vi "Calib_and_iRFAlign_confirm.vi"(6 "Current V":T1, 8 "Ch4 Data":dbl[][](array[numeric]), 9 "Ch3 Data":dbl[][](array[numeric]), 10 "Ch2 Data":dbl[][](array[numeric]), 11 "Ch1 Data":dbl[][](array[numeric])) -> (2 "Save?":bool)   [LabVIEW 2020]
uses:
  GlobalVariables.vi
panel:
  out "Reference Gain":dbl format="%#_3g"
  out "Gain4":dbl format="%#_3g"
  out "Reference V4":dbl format="%#_4g"
  out "Channel 4":dbl[][](graph)
  out "V4":dbl format="%#_4g"
  out "Reference Gain3":dbl format="%#_3g"
  out "Reference Gain 2":dbl format="%#_3g"
  out "Gain3":dbl format="%#_3g"
  out "Gain2":dbl format="%#_3g"
  out "Gain1":dbl format="%#_3g"
  out "Reference Gian1":dbl format="%#_3g"
  out "Reference V3":dbl format="%#_4g"
  out "Reference V2":dbl format="%#_4g"
  out "Reference V1":dbl format="%#_4g"
  in  "Cancel Button":bool
  in  "Save Button":bool
  out "Channel 3":dbl[][](graph)
  out "Channel 2":dbl[][](graph)
  out "Channel 1":dbl[][](graph)
  out "V3":dbl format="%#_4g"
  out "V2":dbl format="%#_4g"
  out "V1":dbl format="%#_4g"
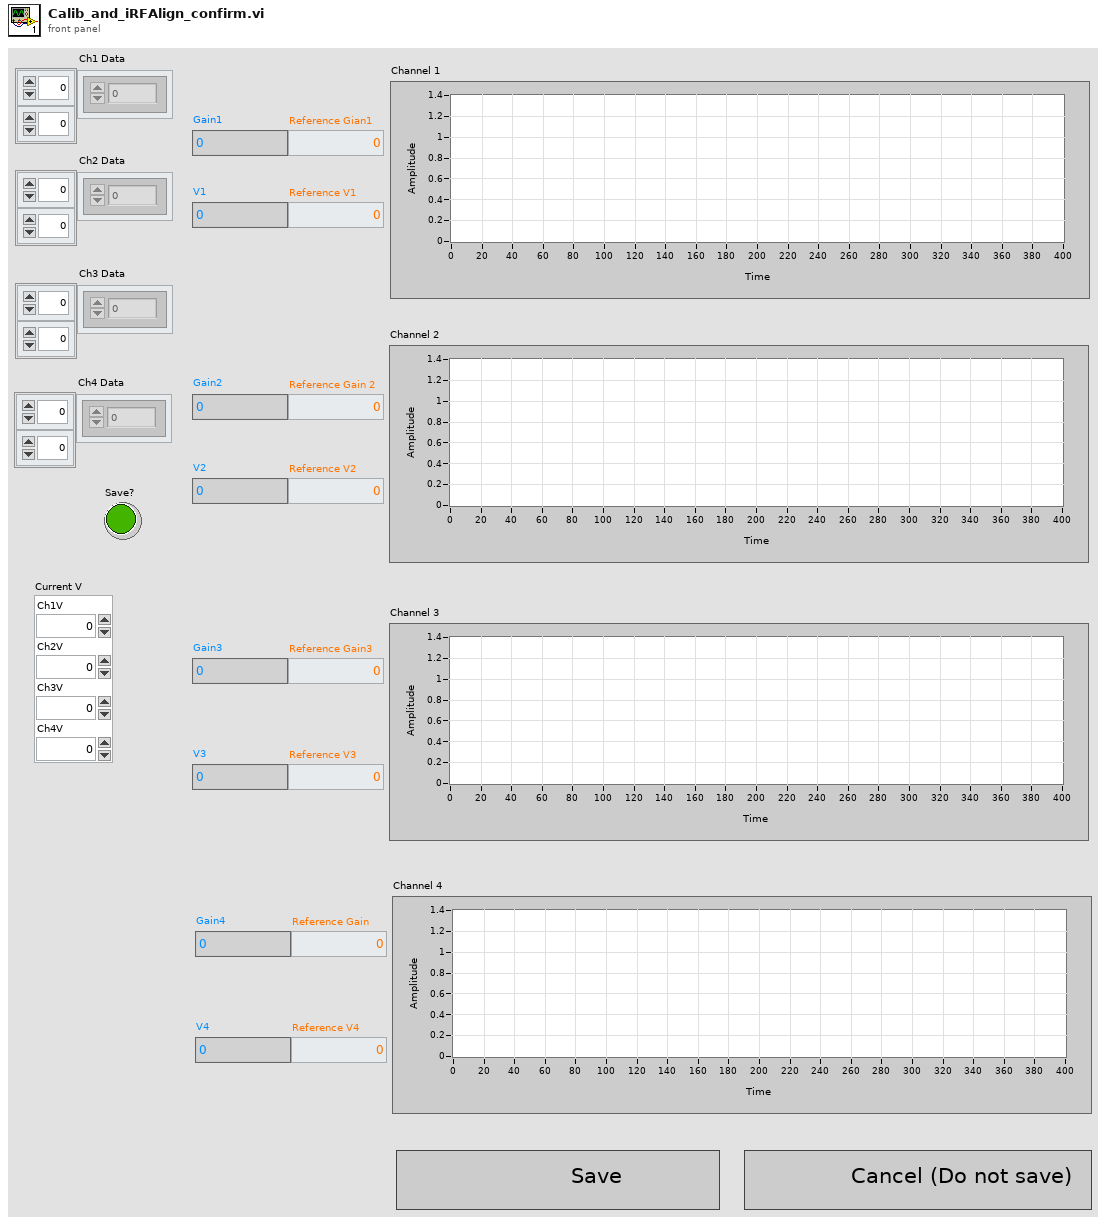
[diagram p1: front panel]
types:
  T1 = cluster{"Ch1V":dbl, "Ch2V":dbl, "Ch3V":dbl, "Ch4V":dbl}
  T2 = cluster{"Ch1 WF":dbl[], "Ch2 WF":dbl[], "Ch3 WF":dbl[], "Ch4 WF":dbl[], "V1":dbl, "V2":dbl, "V3":dbl, "V4":dbl}
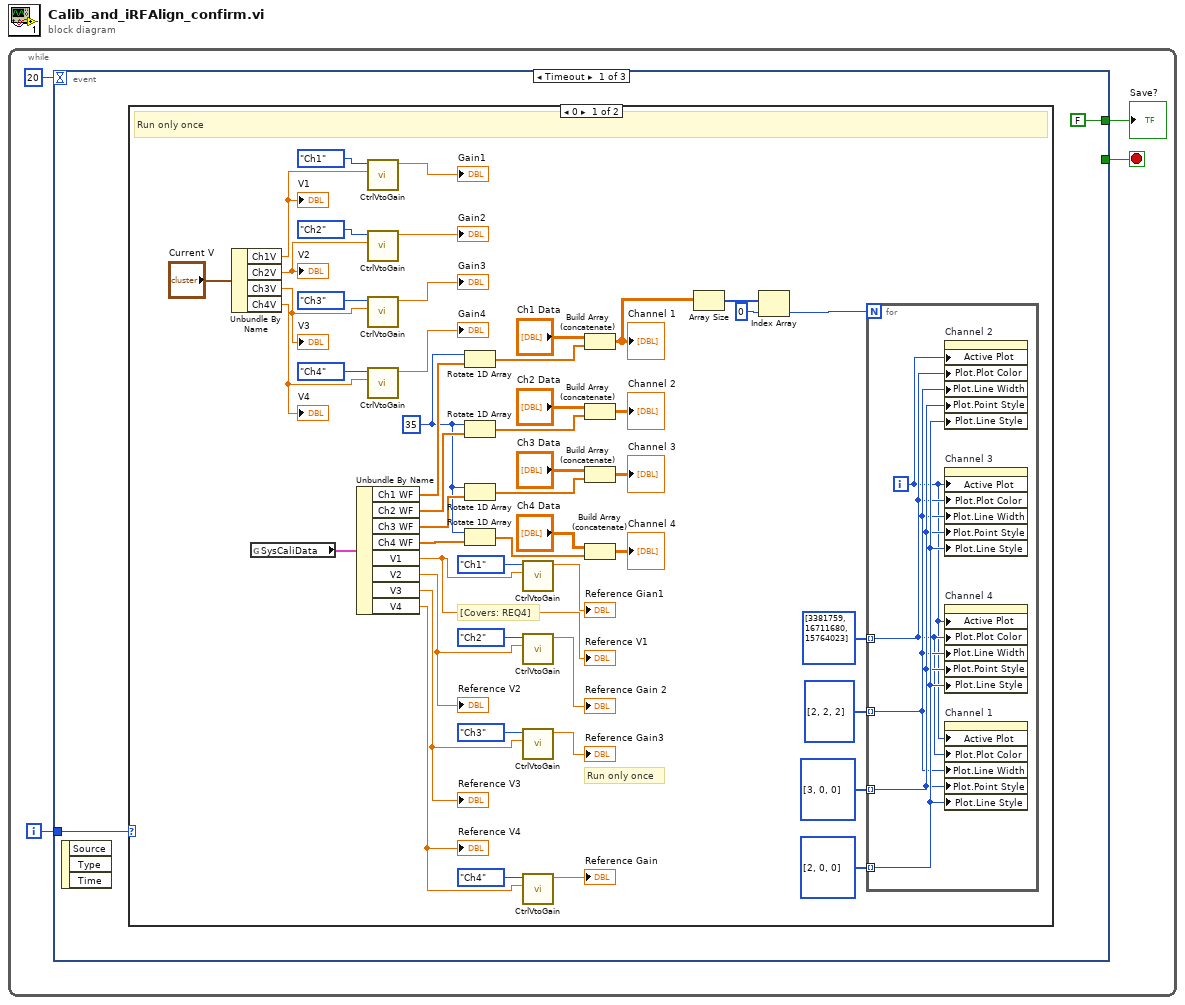
[diagram p0: block diagram]
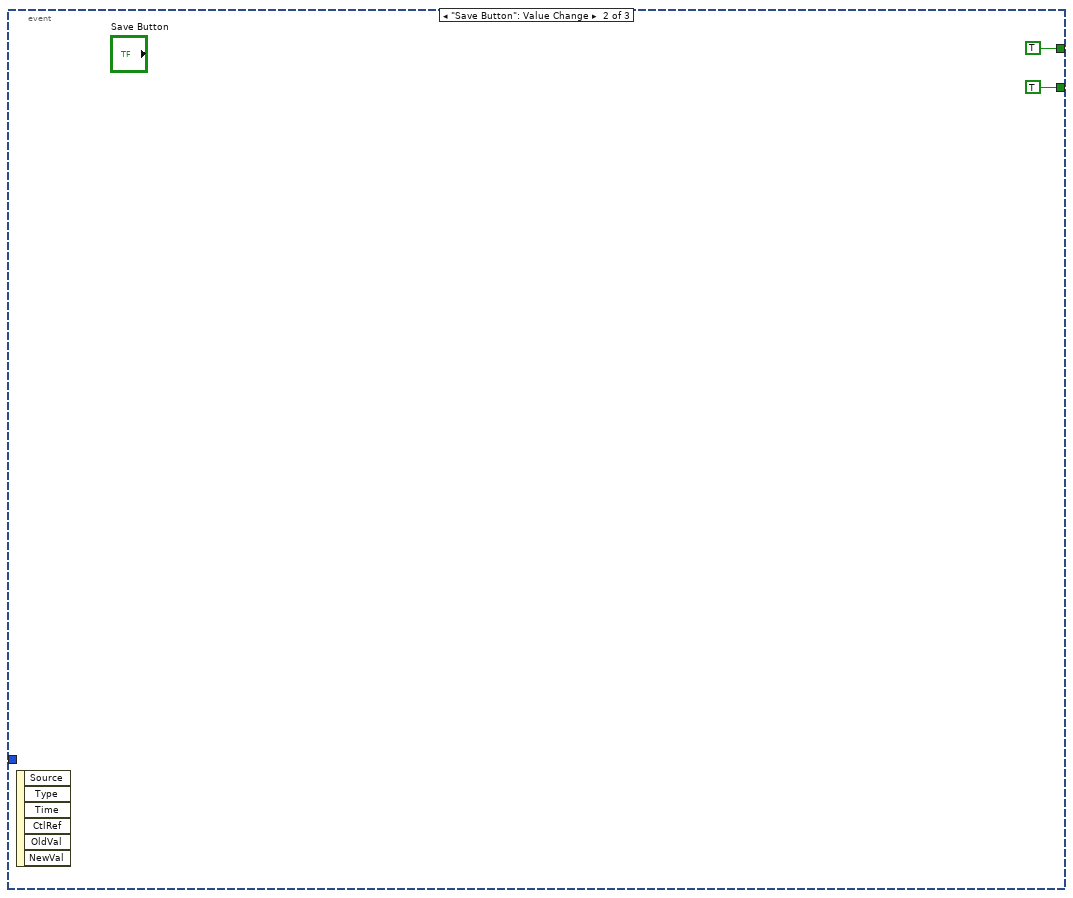
[diagram p3: hidden frame]
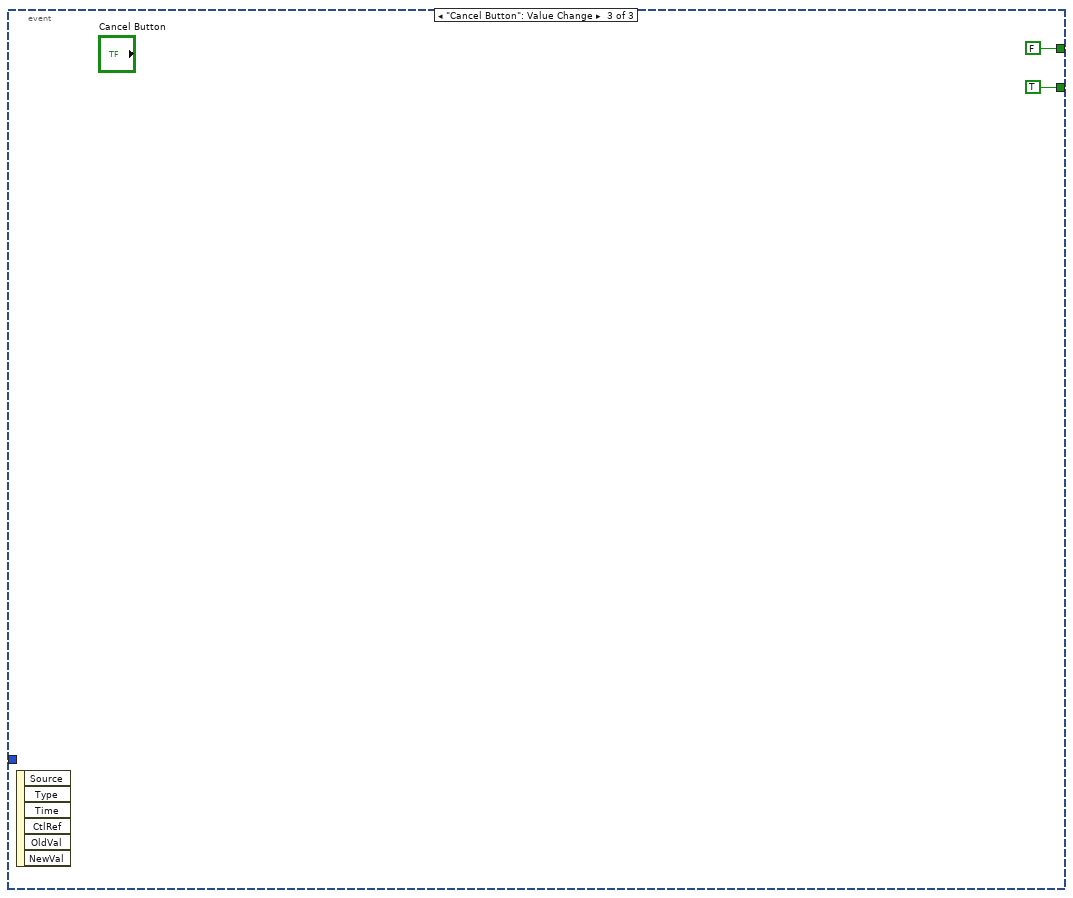
[diagram p4: hidden frame]
diagram:
  n1 = while {
    i -> [w4]
    stop <- w2 stop-if-true
    n2 = event shown="[0] Timeout" {
      selector: _ -> [_ _ _]
      dyn-events: _ -> [_ _ _]
      timeout: 20 -> [_ _ _]
      tunnel: w4 -> [w6 _ _]
      tunnel: [_ TRUE ("Save Button") TRUE ("Save Button")] -> w2
      tunnel: [FALSE ("Save?") TRUE ("Save?") FALSE ("Save?")] -> w1
      event Timeout {
        n3 = event-data() -> ()  [unwired: 1 in, 3 out]
        n4 = case shown="0" w6 {
          frame 0 {
            w23 = 35 ("n")
            # "[Covers: REQ4]"
            # "Run only once"
            # "Run only once"
            n5 = Unbundle By Name("Current V") -> ("Ch1V"=w29:dbl, "Ch2V"=w27:dbl, "Ch3V"=w25:dbl, "Ch4V"=w17:dbl)
            "V1" <- w29
            "V2" <- w27
            "V3" <- w25
            "V4" <- w17
            n6 = global read "GlobalVariables.vi" "SysCaliData"() -> (w54:T2)
            n7 = Unbundle By Name(w54) -> ("Ch1 WF"=w53:dbl[], "Ch2 WF"=w50:dbl[], "Ch3 WF"=w48:dbl[], "Ch4 WF"=w22:dbl[], "V1"=w35:dbl, "V2"=w33:dbl, "V3"=w31:dbl, "V4"=w11:dbl)
            "Reference V1" <- w35
            "Reference V2" <- w33
            "Reference V3" <- w31
            "Reference V4" <- w11
            n8 = call "CtrlVtoGain.vi"("CtrlV(V)"=w29, "Channel"=enum16{"Ch1", "Ch2", "Ch3", "Ch4"}."Ch1") -> ("Gain"=→"Gain1":dbl)  [unwired: 8 in, 1 out]
            n9 = call "CtrlVtoGain.vi"("CtrlV(V)"=w27, "Channel"=enum16{"Ch1", "Ch2", "Ch3", "Ch4"}."Ch2") -> ("Gain"=→"Gain2":dbl)  [unwired: 8 in, 1 out]
            n10 = call "CtrlVtoGain.vi"("CtrlV(V)"=w25, "Channel"=enum16{"Ch1", "Ch2", "Ch3", "Ch4"}."Ch3") -> ("Gain"=→"Gain3":dbl)  [unwired: 8 in, 1 out]
            n11 = call "CtrlVtoGain.vi"("CtrlV(V)"=w17, "Channel"=enum16{"Ch1", "Ch2", "Ch3", "Ch4"}."Ch4") -> ("Gain"=→"Gain4":dbl)  [unwired: 8 in, 1 out]
            n12 = Rotate 1D Array(1:w53, 2:w23) -> (0:w47:dbl[])
            n13 = Rotate 1D Array(1:w50, 2:w23) -> (0:w46:dbl[])
            n14 = Rotate 1D Array(1:w48, 2:w23) -> (0:w45:dbl[])
            n15 = Rotate 1D Array(1:w22, 2:w23) -> (0:w20:dbl[])
            n16 = call "CtrlVtoGain.vi"("CtrlV(V)"=w35, "Channel"=enum16{"Ch1", "Ch2", "Ch3", "Ch4"}."Ch1") -> ("Gain"=→"Reference Gian1":dbl)  [unwired: 8 in, 1 out]
            n17 = call "CtrlVtoGain.vi"("CtrlV(V)"=w33, "Channel"=enum16{"Ch1", "Ch2", "Ch3", "Ch4"}."Ch2") -> ("Gain"=→"Reference Gain 2":dbl)  [unwired: 8 in, 1 out]
            n18 = call "CtrlVtoGain.vi"("CtrlV(V)"=w31, "Channel"=enum16{"Ch1", "Ch2", "Ch3", "Ch4"}."Ch3") -> ("Gain"=→"Reference Gain3":dbl)  [unwired: 8 in, 1 out]
            n19 = call "CtrlVtoGain.vi"("CtrlV(V)"=w11, "Channel"=enum16{"Ch1", "Ch2", "Ch3", "Ch4"}."Ch4") -> ("Gain"=→"Reference Gain":dbl)  [unwired: 8 in, 1 out]
            n20 = Build Array (concatenate)("Ch1 Data", w47) -> (w37:dbl[][])
            "Channel 1" <- w37
            n21 = Build Array (concatenate)("Ch2 Data", w46) -> (→"Channel 2":dbl[][])
            n22 = Build Array (concatenate)("Ch3 Data", w45) -> (→"Channel 3":dbl[][])
            n23 = Build Array (concatenate)("Ch4 Data", w20) -> (→"Channel 4":dbl[][])
            n24 = Array Size(array=w37) -> (size(s)=w43:i32[])
            n25 = Index Array(array=w43, index=0) -> (element=w41:i32)
            n26 = for {
              N: w41 -> [_]
              tunnel: u32[] [3381759, 16711680, 15764023] -> [w58] mode=indexing
              tunnel: i32[] [2, 2, 2] -> [w59] mode=indexing
              tunnel: i32[] [3, 0, 0] -> [w60] mode=indexing
              tunnel: i32[] [2, 0, 0] -> [w61] mode=indexing
              i -> [w57]
              n27 = property on="Channel 2" class="WFGraph (strict)"("Active Plot"=w57, "Plot.Plot Color"=w58, "Plot.Line Width"=w59, "Plot.Point Style"=w60, "Plot.Line Style"=w61) -> ()  [unwired: 2 in, 2 out]
              n28 = property on="Channel 3" class="WFGraph (strict)"("Active Plot"=w57, "Plot.Plot Color"=w58, "Plot.Line Width"=w59, "Plot.Point Style"=w60, "Plot.Line Style"=w61) -> ()  [unwired: 2 in, 2 out]
              n29 = property on="Channel 4" class="WFGraph (strict)"("Active Plot"=w57, "Plot.Plot Color"=w58, "Plot.Line Width"=w59, "Plot.Point Style"=w60, "Plot.Line Style"=w61) -> ()  [unwired: 2 in, 2 out]
              n30 = property on="Channel 1" class="WFGraph (strict)"("Active Plot"=w57, "Plot.Plot Color"=w58, "Plot.Line Width"=w59, "Plot.Point Style"=w60, "Plot.Line Style"=w61) -> ()  [unwired: 2 in, 2 out]
            }
          }
          frame 1, Default {
          }
        }
      }
      event "Save Button": Value Change {
        n31 = event-data() -> ()  [unwired: 1 in, 6 out]
      }
      event "Cancel Button": Value Change {
        n32 = event-data() -> ()  [unwired: 1 in, 6 out]
      }
    }
    "Save?" <- w1
  }
